vi "NPC3SG Get Voltages v10.6.1.vi"(1 "Drive Visa Name":refnum<visa-resource-name>="COM5") -> (0 "Drive Current Voltages":T1 {"Drive Z Voltage" min=-273.0 max=300000.0 step=0.0001 format="%.3f"; "Drive Y Voltage" min=-273.0 max=300000.0 step=0.0001 format="%.3f"; "Drive X Voltage" min=-273.0 max=300000.0 step=0.0001 format="%.3f"})   [LabVIEW 2010]
uses:
  TypeDefs/NPC3SG Current Voltages v10.6.1.ctl
  drivers/Newport NPC3SG/SubNPC3SG.llb/device variables.vi
panel:
  out "Read Error":errorcluster caption="error out" {"code" format="%x"}
  out "Send Error":errorcluster
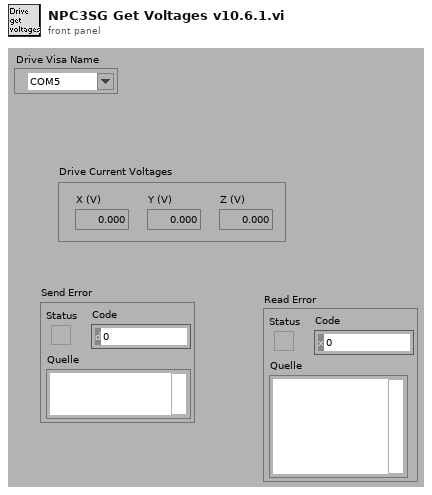
[diagram p1: front panel]
types:
  T1 = typedef "NPC3SG Current Voltages v10.6.1.ctl" = cluster{"Drive X Voltage":dbl, "Drive Y Voltage":dbl, "Drive Z Voltage":dbl}
  T2 = cluster{"Array dc-level open[0]":dbl, "Array dc-level open[1]":dbl, "Array dc-level open[2]":dbl}
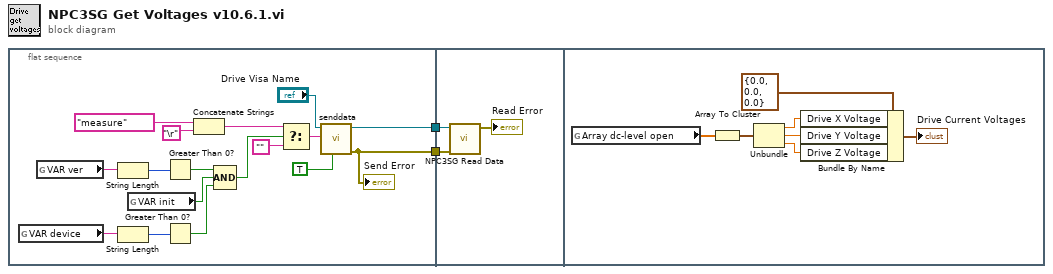
[diagram p0: block diagram]
diagram:
  n1 = flat-sequence {
    tunnel: [w5] -> w2
    tunnel: [w4] -> w1
    tunnel: w2 -> [w20]
    tunnel: w1 -> [w21]
    frame #0 {
      n2 = global read "device variables.vi" "VAR device"() -> (w15:string)
      n3 = global read "device variables.vi" "VAR ver"() -> (w19:string)
      n4 = String Length(string=w19) -> (length=w18:i32)
      n5 = String Length(string=w15) -> (length=w16:i32)
      n6 = global read "device variables.vi" "VAR init"() -> (w17:bool)
      n7 = Greater Than 0?(x=w18) -> (x > 0?=w13:bool)
      n8 = Greater Than 0?(x=w16) -> (x > 0?=w14:bool)
      n9 = Concatenate Strings("measure" ("String"), "\r") -> (w9:string)
      n10 = Compound Arithmetic op=AND(w13, w17, w14) -> (w12:bool)
      n11 = Select(t=w9, s=w12, f="") -> (s? t:f=w7:string)
      n12 = call "senddata.vi"("read ERR"=TRUE, "writebuffer"=w7, "VISA-Ressourcen-Name"="Drive Visa Name") -> ("error out"=w5:errorcluster, "VISA-Ressourcen-Name (Ausgang)"=w4:refnum<visa-resource-name>)  [unwired: 6 in, 1 out]
      "Send Error" <- w5
    }
    frame #1 {
      n13 = call "NPC3SG Read Data.vi"("VISA resource name in"=w21, "error in"=w20) -> ("error ende"=→"Read Error":errorcluster)  [unwired: 8 in]
    }
    frame #2 {
      n14 = global read "device variables.vi" "Array dc-level open"() -> (w27:dbl[])
      n15 = Array To Cluster(array=w27) -> (cluster=w26:T2)
      n16 = Unbundle(w26) -> ("Array dc-level open[0]"=w25:dbl, "Array dc-level open[1]"=w24:dbl, "Array dc-level open[2]"=w23:dbl)
      n17 = Bundle By Name(cluster=T1 {"Drive X Voltage"=0.0, "Drive Y Voltage"=0.0, "Drive Z Voltage"=0.0} ("Drive Current Voltages"), "Drive X Voltage"=w25, "Drive Y Voltage"=w24, "Drive Z Voltage"=w23) -> (→"Drive Current Voltages":T1)
    }
  }
